vi "my RandBeam.vi"(1 "size default 128":i32=128, 2 "重复次数":i32=10) -> (0 "amplitude matrix":cdb[][](array[numeric]))   [LabVIEW 2018]
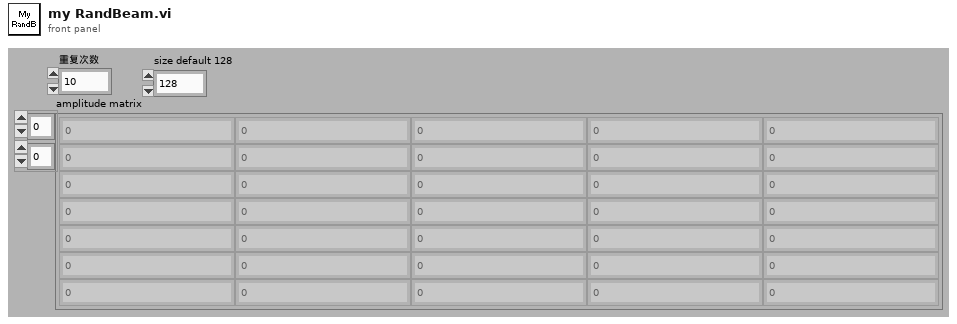
[diagram p1: front panel]
types:
  T1 = cluster{"amplitude matrix":cdb[][], "number of columns in amplitude matrix":i32, "number of rows in amplitude matrix":i32, "represented width (in m)":dbl, "represented height (in m)":dbl, "wavelength (in m)":dbl}
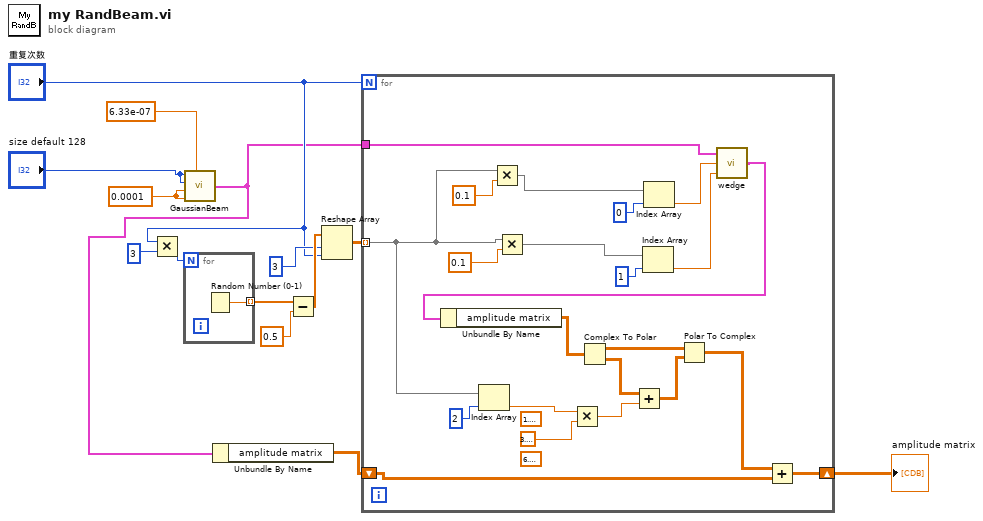
[diagram p0: block diagram]
diagram:
  w12 = 0.0001
  n1 = Multiply(x="重复次数", y=3) -> (x*y=w10:i32)
  n2 = for {
    N: w10 -> [_]
    tunnel: [w15] -> w9 mode=indexing
    n3 = Random Number (0-1)() -> (number: 0 to 1=w15:dbl)
  }
  n4 = call "GaussianBeam.vi"("wavelength (in m; default 633E-9=633nm)"=6.33e-07, "width of represented y range (in m; default 1E-3=1mm)"=w12, "width of represented x range (in m; default 1E-3=1mm)"=w12, "number of rows in amplitude matrix (default 64)"="size default 128", "number of columns in amplitude matrix (default 64)"="size default 128") -> ("Gaussian beam"=w3:T1)  [unwired: 1 in]
  n5 = Unbundle By Name(w3) -> ("amplitude matrix"=w2:cdb[][])
  n6 = Subtract(x=w9, y=0.5) -> (x-y=w7:dbl[])
  n7 = Reshape Array(w7, 3, "重复次数") -> (w5:dbl[][])
  n8 = for {
    N: "重复次数" -> [_]
    tunnel: w5 -> [w17] mode=indexing
    shift-right: [w24] -> w1
    shift-left: w2 -> [w30]
    tunnel: w3 -> [w26]
    (unwired) 1.5707963267948966
    (unwired) 6.283185307179586
    n9 = Index Array(array=w17, index=2) -> (element=w33:dbl)
    n10 = Multiply(x=w17, y=0.1) -> (x*y=w18:dbl[])
    n11 = Multiply(x=w17, y=0.1) -> (x*y=w36:dbl[])
    n12 = Multiply(x=w33, y=3.141592653589793) -> (x*y=w32:dbl)
    n13 = Index Array(array=w36, index=1) -> (element=w28:dbl)
    n14 = Index Array(array=w18, index=0) -> (element=w29:dbl)
    n15 = call "wedge.vi"("angle in y-z plane, beta"=w28, "angle in x-z plane, alpha"=w29, "beam in front of spiral wave plate"=w26) -> ("beam behind spiral wave plate"=w20:T1)
    n16 = Unbundle By Name(w20) -> ("amplitude matrix"=w21:cdb[][])
    n17 = Complex To Polar(r * e^(i*theta)=w21) -> (r=w31:dbl[][], theta=w23:dbl[][])
    n18 = Add(x=w23, y=w32) -> (x+y=w22:dbl[][])
    n19 = Polar To Complex(1:w22, 2:w31) -> (0:w25:cdb[][])
    n20 = Add(x=w25, y=w30) -> (x+y=w24:cdb[][])
  }
  "amplitude matrix" <- w1
